vi "State7-Parked.vi"(11 "Boolean in":refnum<vi>) -> (1 "Cluster":T2, 2 "Front/Back 2":enum16{"Forward", "Backward", "Stop"}(ring), 3 "Left/Right":enum16{"Left", "Right", "Stop"}(ring), 4 "Enum":T1, 5 "Back Speed":u32, 6 "Left/Right Speed":u32)   [LabVIEW 2014]
uses:
  FPGA Bitfiles/Parking States Indicators.ctl
  FPGA Bitfiles/Parking States.ctl
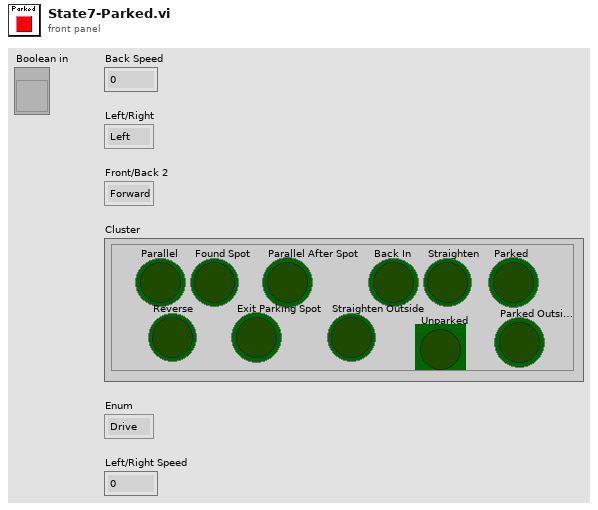
[diagram p1: front panel]
types:
  T1 = typedef "Parking States.ctl" = enum16{"Drive", "Parallel", "Found Spot", "Parallel After Spot", "Back In", "Straighten", "Parked", "Reverse", "Exit Parking Spot", "Straighten Outside", "Unparked", "Parked Outside"}
  T2 = typedef "Parking States Indicators.ctl" = cluster{"Parallel":bool, "Found Spot":bool, "Parallel After Spot":bool, "Back In":bool, "Straighten":bool, "Parked":bool, "Reverse":bool, "Exit Parking Spot":bool, "Straighten Outside":bool, "Unparked":bool, "Parked Outside":bool}
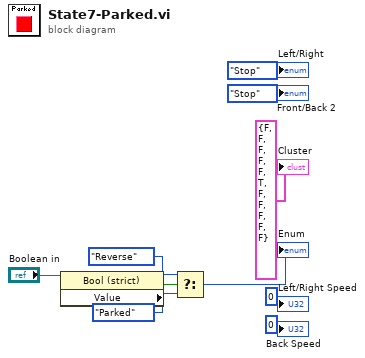
[diagram p0: block diagram]
diagram:
  n1 = property class="Bool (strict)"(reference="Boolean in") -> ("Value"=w6:bool)  [unwired: 1 in, 2 out]
  n2 = Select(t=Parking_States."Reverse", s=w6, f=Parking_States."Parked") -> (s? t:f=→"Enum":T1)
  "Cluster" <- T2 {"Parallel"=FALSE, "Found Spot"=FALSE, "Parallel After Spot"=FALSE, "Back In"=FALSE, "Straighten"=FALSE, "Parked"=TRUE, "Reverse"=FALSE, "Exit Parking Spot"=FALSE, "Straighten Outside"=FALSE, "Unparked"=FALSE, "Parked Outside"=FALSE} ("Cluster")
  "Back Speed" <- u32 0 ("Back Speed")
  "Front/Back 2" <- enum16{"Forward", "Backward", "Stop"}."Stop" ("Front/Back 2")
  "Left/Right" <- enum16{"Left", "Right", "Stop"}."Stop" ("Left/Right")
  "Left/Right Speed" <- u32 0 ("Left/Right Speed")
